vi "Defer Panel Updates.vi"() -> ()   [LabVIEW 2012]
panel:
  in  "延迟前面板更新":bool
  in  "停止按钮":bool
  in  "已禁用状态":T1(ring)
  out "波形图表2":dbl(graph)
  in  "温度计2":dbl(slide) scale=0.0..100.0
  in  "垂直填充滑动杆2":dbl(slide) scale=0.0..10.0
  in  "暂停按钮2":bool
  in  "弹出按钮2":bool
  in  "帮助按钮2":bool
  in  "向下按钮2":bool
  in  "复制按钮2":bool
  in  "播放按钮2":bool
  in  "邮件按钮2":bool
  in  "打开按钮2":bool
  in  "添加按钮2":bool
  in  "新建按钮2":bool
  in  "向上按钮2":bool
  in  "确定按钮2":bool
  out "波形图表":dbl(graph)
  in  "温度计":dbl(slide) scale=0.0..100.0
  in  "垂直填充滑动杆":dbl(slide) scale=0.0..10.0
  in  "暂停按钮":bool
  in  "弹出按钮":bool
  in  "帮助按钮":bool
  in  "向下按钮":bool
  in  "复制按钮":bool
  in  "播放按钮":bool
  in  "邮件按钮":bool
  in  "打开按钮":bool
  in  "添加按钮":bool
  in  "新建按钮":bool
  in  "向上按钮":bool
  in  "确定按钮":bool
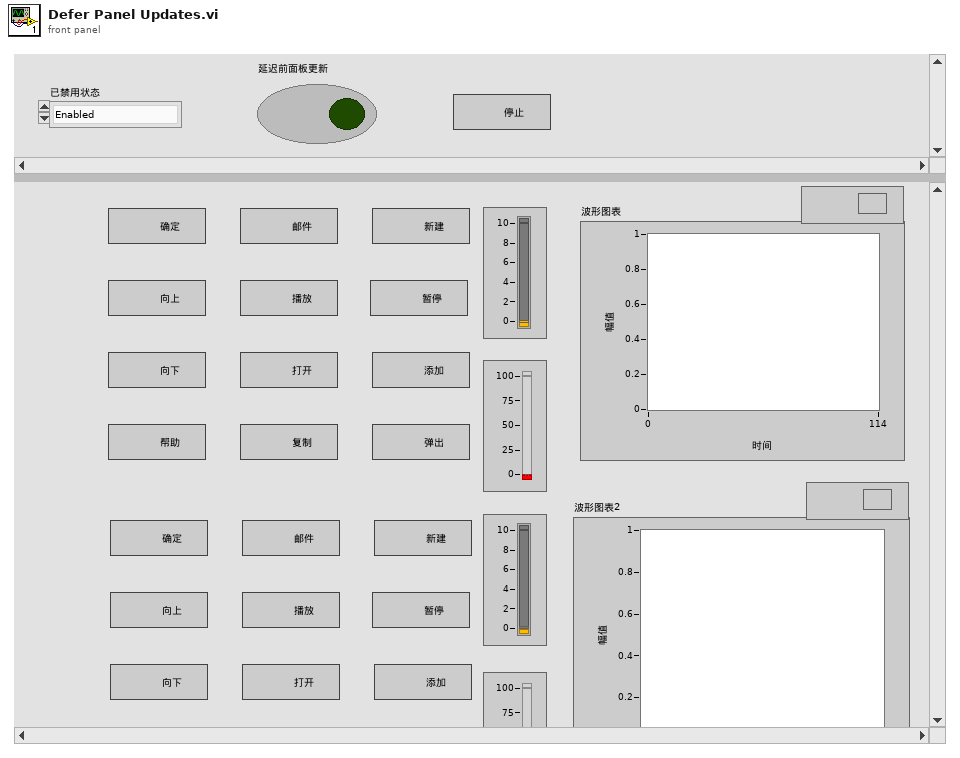
[diagram p1: front panel]
types:
  T1 = enum8{"Enabled", "Disabled", "Disabled and Grayed Out"}
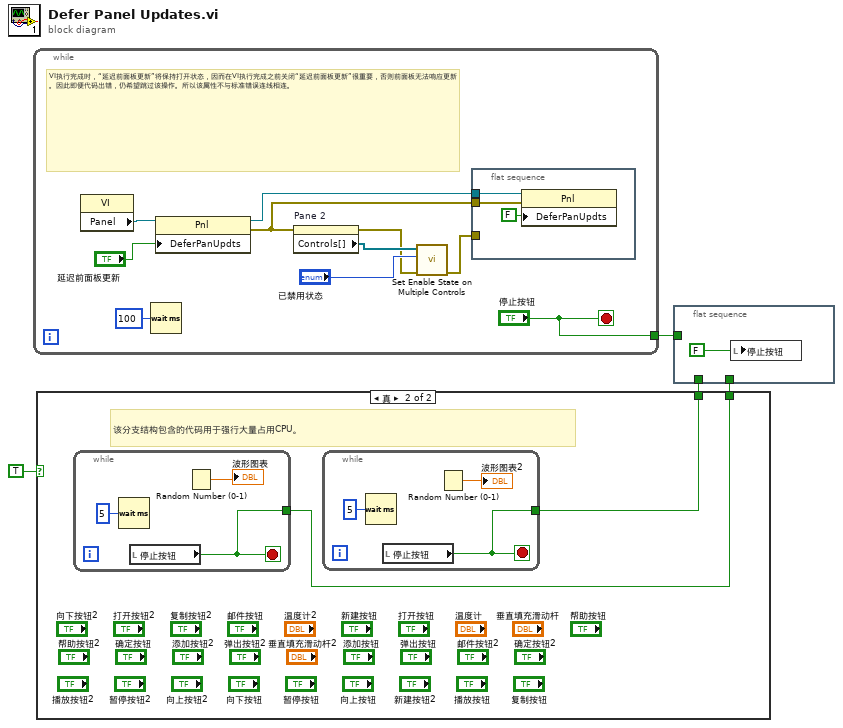
[diagram p0: block diagram]
diagram:
  n1 = while {
    tunnel: ["停止按钮"] -> w4
    stop <- "停止按钮" stop-if-true
    # "VI执行完成时，“延迟前面板更新”将保持打开状态，因而在VI执行完成之前关闭“延迟前面板更新”很重要，否则前面板无法响应更新。因此即便代码出错，仍希望跳过该操作。所以该属性不与标准错误连线相连。"
    n2 = property on="属性节点" class="VI"() -> ("Panel"=w8:refnum<vi>)  [unwired: 2 in, 2 out]
    n3 = Wait (ms) ("等待(ms)")(milliseconds to wait=u32 100 ("等待时间（毫秒）")) -> ()  [unwired: 1 out]
    n4 = property on="属性节点" class="Pnl"(reference=w8, "DeferPanUpdts"="延迟前面板更新") -> (reference out=w7:refnum<vi>, error out=w10:errorcluster)  [unwired: 1 in]
    n5 = property on="Pane 2" class="Pane"(error in=w10) -> (error out=w11:errorcluster, "Controls[]"=w12:refnum<vi>[])  [unwired: 1 in, 1 out]
    n6 = call "Set Enable State on Multiple Controls.vi"("错误输入"=w11, "已禁用状态"="已禁用状态", "控件"=w12) -> ("错误输出"=w9:cluster{"状态":bool, "代码":i32, "源":string})  [unwired: 8 in]
    n7 = flat-sequence {
      tunnel: w10 -> [w16]
      tunnel: w9 -> [_]
      tunnel: w7 -> [w15]
      frame #0 {
        n8 = property on="属性节点" class="Pnl"(reference=w15, error in=w16, "DeferPanUpdts"=FALSE ("延迟前面板更新")) -> ()  [unwired: 2 out]
      }
    }
  }
  n9 = case shown="真" TRUE {
    tunnel: [_ w19] -> w2
    tunnel: [_ w18] -> w1
    frame False {
    }
    frame True {
      # "该分支结构包含的代码用于强行大量占用CPU。"
      n10 = while {
        tunnel: [w25] -> w18
        stop <- w25 stop-if-true
        n11 = Wait (ms) ("等待(ms)")(milliseconds to wait=u32 5 ("等待时间（毫秒）")) -> ()  [unwired: 1 out]
        n12 = local read "停止按钮"() -> (w25:bool)
        n13 = Random Number (0-1) ("随机数(0-1)")() -> (number: 0 to 1=→"波形图表":dbl)
      }
      n14 = while {
        tunnel: [w22] -> w19
        stop <- w22 stop-if-true
        n15 = Wait (ms) ("等待(ms)")(milliseconds to wait=u32 5 ("等待时间（毫秒）")) -> ()  [unwired: 1 out]
        n16 = local read "停止按钮"() -> (w22:bool)
        n17 = Random Number (0-1) ("随机数(0-1)")() -> (number: 0 to 1=→"波形图表2":dbl)
      }
    }
  }
  n18 = flat-sequence {
    tunnel: w4 -> [_]
    tunnel: w2 -> [_]
    tunnel: w1 -> [_]
    frame #0 {
      n19 = local write "停止按钮"(FALSE ("停止按钮")) -> ()
    }
  }
